vi "obj_area.vi"() -> ()   [LabVIEW 2022 SP3]
panel:
  out "XY Graph 2":cluster{cdb[]}[](graph)
  out "Array 4":string[](array[string])
  out "input_camera":string[](array[string])
  out "joint=":string[](array[string])
  out "input_radar":string[](array[string])
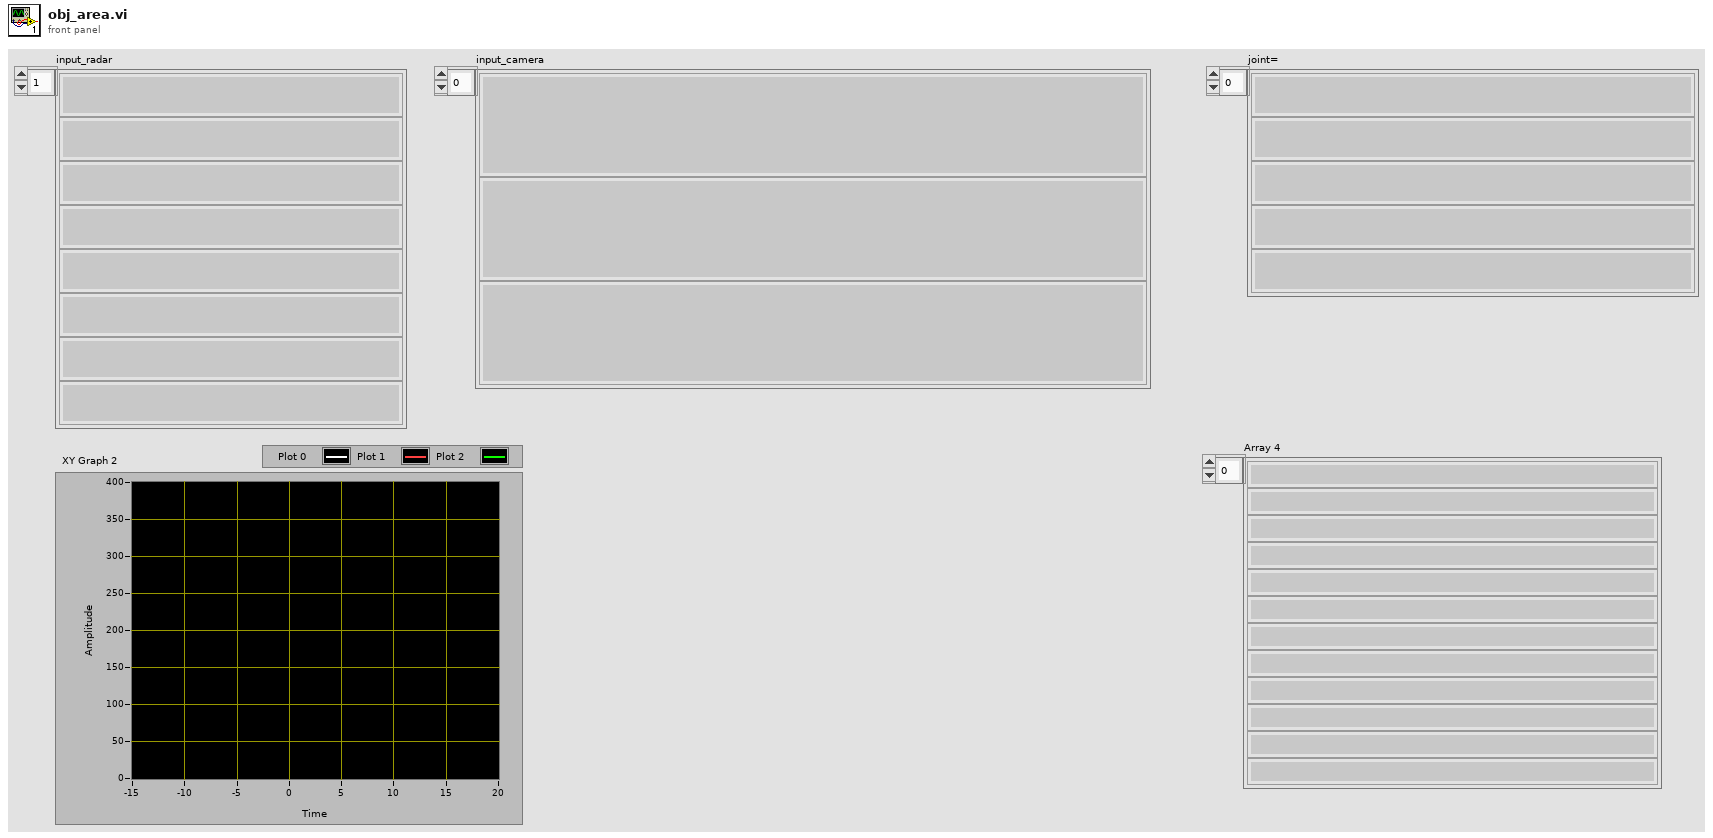
[diagram p1: front panel]
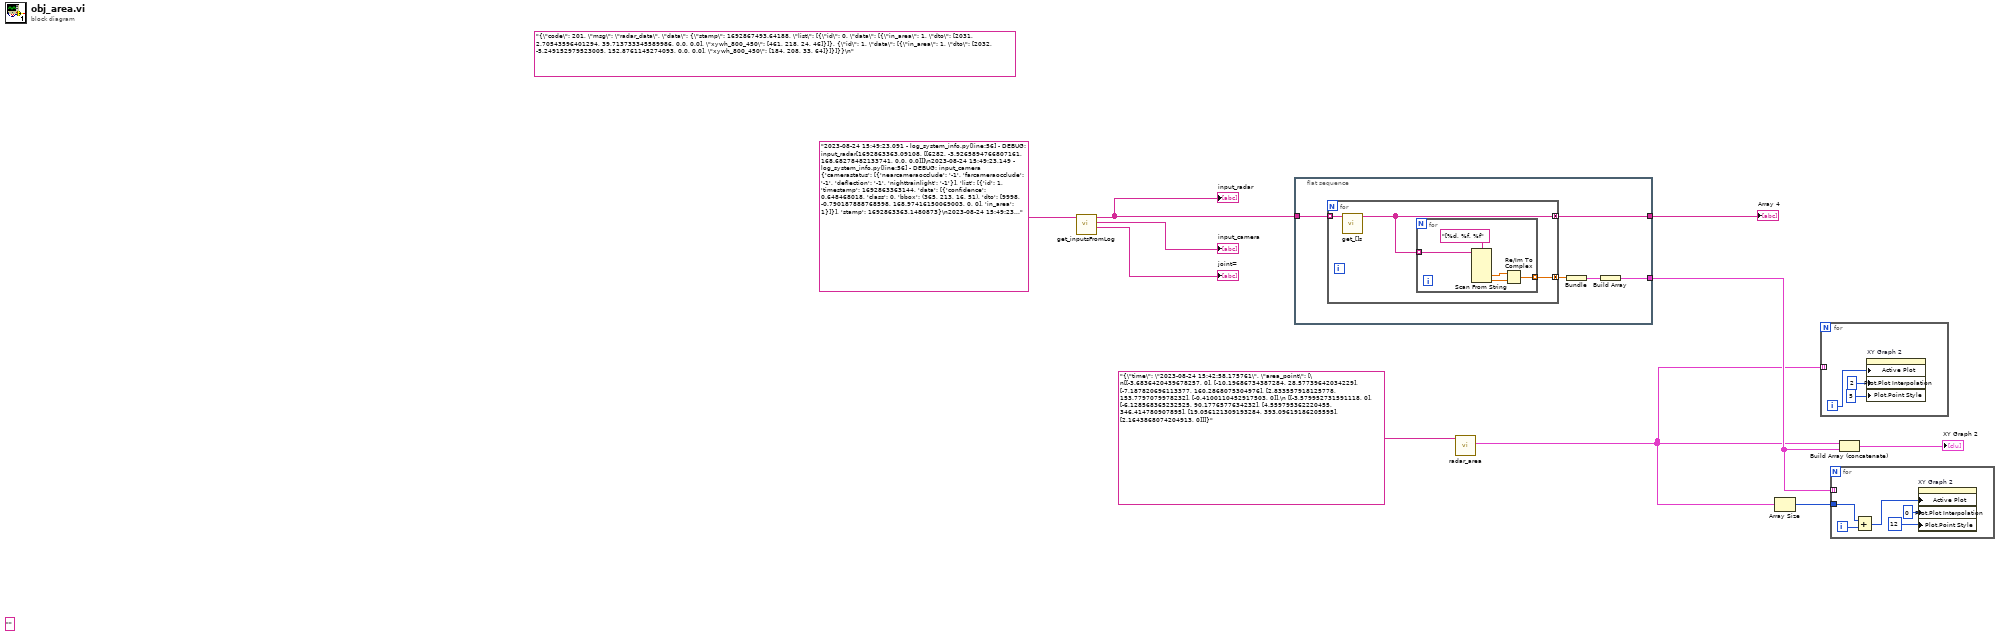
[diagram p0: block diagram]
diagram:
  (unwired) "" ("112_radar_area")
  (unwired) "{\"code\": 201, \"msg\": \"radar_data\", \"data\": {\"stamp\": 1692867493.64188, \"list\": [{\"id\": 0, \"data\": [{\"in_area\": 1, \"dto\": [2031, 2.70543596401294, 39.713733345589986, 0.0, 0.0], \"xywh_800_450\": [461, 218, 24, 46]}]}, {\"id\": 1, \"data\": [{\"in_area\": 1, \"dto\": [2032, -5.249152979523005, 152.8761145274093, 0.0, 0.0], \"xywh_800_450\": [184, 208, 33, 64]}]}]}}\n"
  n1 = call "get_inputsFromLog.vi"("String"="2023-08-24 15:49:23,091 - log_system_info.py[line:56] - DEBUG: input_radar[1692863363.09108, [[6282, -3.9265894766807161, 168.68278482133741, 0.0, 0.0]]]\n2023-08-24 15:49:23,149 - log_system_info.py[line:56] - DEBUG: input_camera {'camerastatus': [{'nearcameraocclude': '-1', 'farcameraocclude': '-1', 'deflection': '-1', 'nighttrainlight': '-1'}], 'list': [{'id': 1, 'timestamp': 1692863363144, 'data': [{'confidence': 0.648468018, 'class': 0, 'bbox': (365, 213, 16, 51), 'dto': [9998, -0.790187888768598, 168.97416150069003, 0, 0], 'in_area': 1}]}], 'stamp': 1692863363.1480873}\n2023-08-24 15:49:23,170 - log_system_info.py[line:56] - DEBUG: camera=1.23/20,move_coefficient=1.00,radar=0.00/45, joint=0.0/150,block=0,alarm=0\n2023-08-24 15:49:23,218 - log_system_info.py[line:56] - DEBUG: input_radar[1692863363.218035, [[6282, -3.8256106810999433, 168.4832772203718, 0.0, 0.0]]]\n2023-08-24 15:49:23,345 - log_system_info.py[line:56] - DEBUG: input_radar[1692863363.345177, [[6282, -3.72463188551917, 168.2837696194062, 0.0, 0.0]]]\n2023-08-24 15:49:23,349 - log_system_info.py[line:56] - DEBUG: input_camera {'camerastatus': [{'nearcameraocclude': '-1', 'farcameraocclude': '-1', 'deflection': '-1', 'nighttrainlight': '-1'}], 'list': [{'id': 1, 'timestamp': 1692863363344, 'data': [{'confidence': 0.639858961, 'class': 0, 'bbox': (366, 213, 15, 51), 'dto': [9998, -0.7755548834418494, 168.97416150069003, 0, 0], 'in_area': 1}]}], 'stamp': 1692863363.3482804}\n2023-08-24 15:49:23,423 - log_system_info.py[line:56] - DEBUG: camera=2.43/20,move_coefficient=1.00,radar=0.00/45, joint=0.0/150,block=0,alarm=0\n2023-08-24 15:49:23,473 - log_system_info.py[line:56] - DEBUG: input_radar[1692863363.472982, [[6282, -3.7265918776759124, 168.68376481741578, 0.0, 0.0]]]\n2023-08-24 15:49:23,550 - log_system_info.py[line:56] - DEBUG: input_camera {'camerastatus': [{'nearcameraocclude': '-1', 'farcameraocclude': '-1', 'deflection': '-1', 'nighttrainlight': '-1'}], 'list': [{'id': 1, 'timestamp': 1692863363545, 'data': [{'confidence': 0.715841651, 'class': 0, 'bbox': (363, 211, 18, 55), 'dto': [9998, -0.7999404189240135, 164.95041952224807, 0, 0], 'in_area': 1}]}], 'stamp': 1692863363.5489688}\n2023-08-24 15:49:23,599 - log_system_info.py[line:56] - DEBUG: input_radar[1692863363.5992825, [[6282, -3.6285530703302529, 169.08425001346458, 0.0, 0.0]]]\n2023-08-24 15:49:23,675 - log_system_info.py[line:56] - DEBUG: camera=7.59/20,move_coefficient=1.00,radar=0.00/45, joint=0.0/150,block=0,alarm=0\n2023-08-24 15:49:23,733 - log_system_info.py[line:56] - DEBUG: input_radar[1692863363.7334256, [[6282, -3.5305142629845938, 169.48473520951339, 0.0, 0.0]]]\n2023-08-24 15:49:23,757 - log_system_info.py[line:56] - DEBUG: input_camera {'camerastatus': [{'nearcameraocclude': '-1', 'farcameraocclude': '-1', 'deflection': '-1', 'nighttrainlight': '-1'}], 'list': [{'id': 1, 'timestamp': 1692863363746, 'data': [{'confidence': 0.787980318, 'class': 0, 'bbox': (366, 213, 16, 53), 'dto': [9998, -0.7428022186624417, 164.95041952224807, 0, 0], 'in_area': 1}]}], 'stamp': 1692863363.7558203}\n2023-08-24 15:49:23,855 - log_system_info.py[line:56] - DEBUG: input_radar[1692863363.8554313, [[6282, -3.6314930585653671, 169.68424281047899, 0.0, 0.0]]]\n2023-08-24 15:49:23,927 - log_system_info.py[line:56] - DEBUG: camera=13.98/20,move_coefficient=1.00,radar=0.00/45, joint=0.0/150,block=0,alarm=0\n2023-08-24 15:49:23,949 - log_system_info.py[line:56] - DEBUG: input_camera {'camerastatus': [{'nearcameraocclude': '-1', 'farcameraocclude': '-1', 'deflection': '-1', 'nighttrainlight': '-1'}], 'list': [{'id': 1, 'timestamp': 1692863363944, 'data': [{'confidence': 0.831088424, 'class': 0, 'bbox': (365, 211, 17, 52), 'dto': [9998, -0.7851309148955614, 171.06054109798455, 0, 0], 'in_area': 1}]}], 'stamp': 1692863363.9486346}\n2023-08-24 15:49:23,986 - log_system_info.py[line:56] - DEBUG: input_radar[1692863363.9866192, [[6282, -3.533454251219708, 170.0847280065278, 0.0, 0.0]]]") -> ("joint="=→"joint=":string[], "input_camera"=→"input_camera":string[], "Array"=w8:string[])  [unwired: 8 in]
  "input_radar" <- w8
  n2 = flat-sequence {
    tunnel: w8 -> [w15]
    tunnel: [w13] -> w4
    tunnel: [w11] -> w1
    frame #0 {
      n3 = for {
        tunnel: w15 -> [w18] mode=indexing
        tunnel: [w17] -> w11 mode=concatenating
        tunnel: [w16] -> w12 mode=concatenating
        n4 = call "get_[]s.vi"("String"=w18) -> ("[]Array"=w17:string[])  [unwired: 10 in]
        n5 = for {
          tunnel: w17 -> [w23] mode=indexing
          tunnel: [w19] -> w16 mode=indexing
          n6 = Scan From String(format string="[%d, %f, %f", input string=w23) -> (output 2=w20:dbl, output 3=w21:dbl)  [unwired: 6 in, 3 out]
          n7 = Re/Im To Complex(1:w21, 2:w20) -> (0:w19:cdb)
        }
      }
      n8 = Bundle(w12) -> (w14:cluster{cdb[]})  [unwired: 1 in]
      n9 = Build Array(w14) -> (w13:cluster{cdb[]}[])
    }
  }
  n10 = call "radar_area.vi"("String"="{\"time\": \"2023-08-24 15:42:58.175761\", \"area_point\": [\n[[-3.6836420439678257, 0], [-10.19686734387284, 28.57739642034229], [-7.187820696113377, 160.2868075304976], [2.833557918125778, 153.7797079978232], [-0.4100110452917503, 0]],\n [[-3.579952731591118, 0], [-6.128568365232525, 90.1776577634232], [4.559795362220455, 346.414780907895], [19.056121309193284, 393.09619186205595], [2.1643868074204913, 0]]]}") -> ("area point Array"=w2:cluster{cdb[]}[])  [unwired: 9 in, 1 out]
  n11 = Array Size(array=w2) -> (size(s)=w5:i32)
  n12 = for {
    tunnel: w2 -> [_] mode=indexing
    i -> [w24]
    n13 = property on="XY Graph 2" class="XYGraph (strict)"("Active Plot"=w24, "Plot.Plot Interpolation"=u8 2, "Plot.Point Style"=u8 5) -> ()  [unwired: 2 in, 2 out]
  }
  n14 = for {
    tunnel: w5 -> [w30]
    tunnel: w4 -> [_] mode=indexing
    i -> [w31]
    n15 = Add(x=w30, y=w31) -> (x+y=w29:i32)
    n16 = property on="XY Graph 2" class="XYGraph (strict)"("Active Plot"=w29, "Plot.Plot Interpolation"=u8 0, "Plot.Point Style"=u8 12 ("Plot.Plot Interpolation")) -> ()  [unwired: 2 in, 2 out]
  }
  n17 = Build Array (concatenate)(w2, w4) -> (→"XY Graph 2":cluster{cdb[]}[])
  "Array 4" <- w1
